vi "Load Variant Data To OI.vi"(8 "error in (no error)":errorcluster, 11 "TS UI Data in":T1) -> (0 "error out":errorcluster)   [LabVIEW 2015]
uses:
  Type defs/TS UI Data.ctl
  Type defs/Nest cluster.ctl
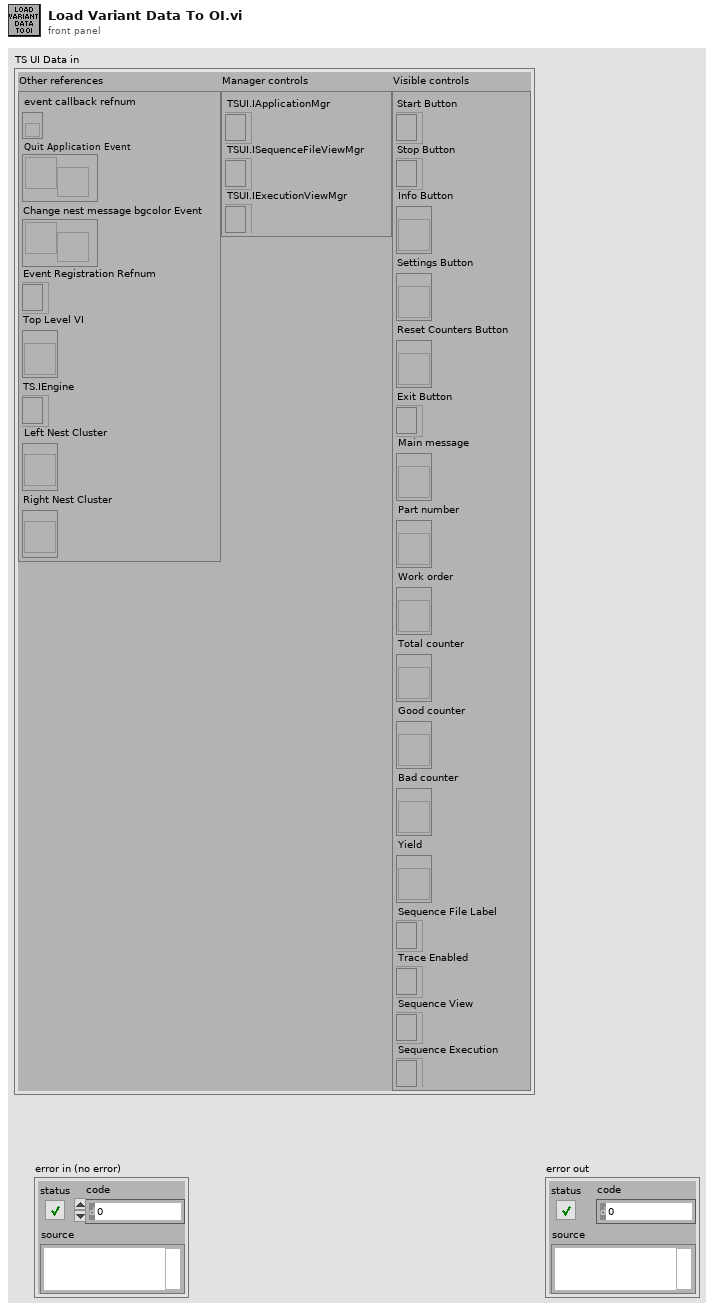
[diagram p1: front panel]
types:
  T1 = typedef "TS UI Data.ctl" = cluster{"Other references":cluster{"event callback refnum":refnum<k27>, "Quit Application Event":refnum<user-event>, "Change nest message bgcolor Event":refnum<user-event>, "event registration refnum":refnum<event-registration>, "Top Level VI":refnum<vi>, "TS.IEngine":refnum<k7>, "Left Nest Cluster":refnum<vi>, "Right Nest Cluster":refnum<vi>}, "Manager controls":cluster{"TSUI.IApplicationMgr":refnum<k7>, "TSUI.ISequenceFileViewMgr":refnum<k7>, "TSUI.IExecutionViewMgr":refnum<k7>}, "Visible controls":cluster{"Start Button":refnum<k7>, "Stop Button":refnum<k7>, "Info Button":refnum<vi>, "Settings Button":refnum<vi>, "Reset Counters Button":refnum<vi>, "Exit Button":refnum<k7>, "Main message":refnum<vi>, "Part number":refnum<vi>, "Work order":refnum<vi>, "Total counter":refnum<vi>, "Good counter":refnum<vi>, "Bad counter":refnum<vi>, "Yield":refnum<vi>, "Sequence File Label":refnum<k7>, "Trace Enabled":refnum<k7>, "Sequence View":refnum<k7>, "Sequence Execution":refnum<k7>}}
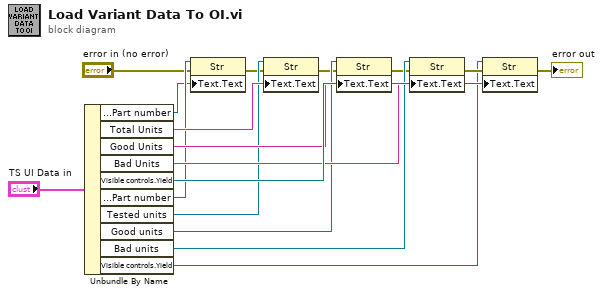
[diagram p0: block diagram]
diagram:
  n1 = Unbundle By Name("TS UI Data in") -> ("Visible controls.Part number"=w3:refnum<vi>, "Total Units"=w14:string, "Good Units"=w15:string, "Bad Units"=w16:string, "Visible controls.Yield"=w17:refnum<vi>, "Visible controls.Part number"=w7:refnum<vi>, "Tested units"=w8:refnum<vi>, "Good units"=w9:refnum<vi>, "Bad units"=w10:refnum<vi>, "Visible controls.Yield"=w11:refnum<vi>)
  n2 = property class="Str"(reference=w7, error in="error in (no error)", "Text.Text"=w3) -> (error out=w4:errorcluster)  [unwired: 1 out]
  n3 = property class="Str"(reference=w8, error in=w4, "Text.Text"=w14) -> (error out=w5:errorcluster)  [unwired: 1 out]
  n4 = property class="Str"(reference=w9, error in=w5, "Text.Text"=w15) -> (error out=w6:errorcluster)  [unwired: 1 out]
  n5 = property class="Str"(reference=w10, error in=w6, "Text.Text"=w16) -> (error out=w12:errorcluster)  [unwired: 1 out]
  n6 = property class="Str"(reference=w11, error in=w12, "Text.Text"=w17) -> (error out=→"error out":errorcluster)  [unwired: 1 out]
